vi "0-Write MDF.vi"(3 "error in":errorcluster, 4 "Global No Sail Circles":T2[](array[typedef]), 5 "Missions (Object Array)":refnum<class "GenericMission.lvclass">[](array[class])) -> (0 "error out":errorcluster)   [LabVIEW 2011]
doc: "Saves a MDF (Mission Definition File) to be later opened by 0-Read MDF.vi. MDF contains mission data: currently only a list of waypoints. The file uses the LabVIEW XML Schema."
uses:
  2-Think/2 Classes/Missions/GenericMission/GenericMission.lvclass
  2-Think/2 Typedefs/UTM Circle.ctl
  0 Typedefs/MDF data cluster.ctl
panel:
  out "MDF data cluster":T1
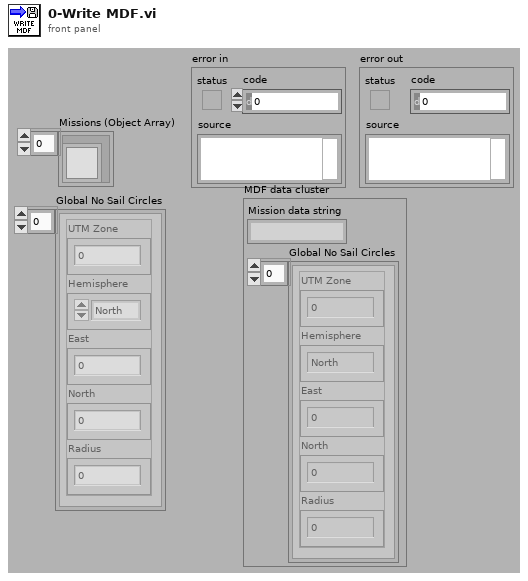
[diagram p1: front panel]
types:
  T1 = typedef "MDF data cluster.ctl" = cluster{"Mission data string":string, "Global No Sail Circles":T2[]}
  T2 = typedef "UTM Circle.ctl" = cluster{"UTM Zone":dbl, "Hemisphere":enum16{"North", "South"}, "East":dbl, "North":dbl, "Radius":dbl}
  T3 = cluster{"data string":string, "Global No Sail Circles":T2[]}
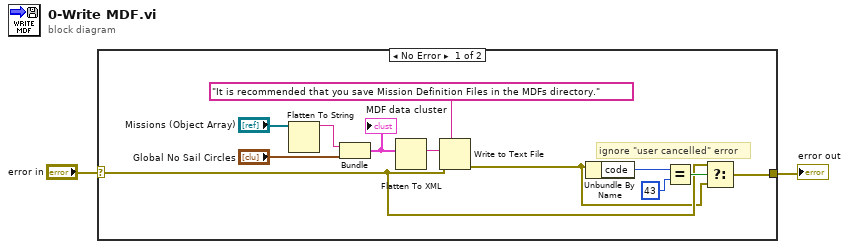
[diagram p0: block diagram]
diagram:
  n1 = case shown="No Error" "error in" {
    selector: "error in" -> [w9 w15]
    tunnel: [w7 w15] -> w1
    frame No Error {
      # "ignore \"user cancelled\" error"
      n2 = Flatten To String(anything="Missions (Object Array)") -> (data string=w5:string)  [unwired: 3 in, 2 out]
      n3 = Bundle("data string"=w5, "Global No Sail Circles"="Global No Sail Circles") -> (w6:T3)  [unwired: 1 in]
      "MDF data cluster" <- w6
      n4 = Flatten To XML(anything=w6) -> (xml string=w14:string)
      n5 = Write to Text File(prompt (Choose or enter file path)="It is recommended that you save Mission Definition Files in the MDFs directory.", text=w14, error in=w9) -> (error out=w8:errorcluster)  [unwired: 1 in, 2 out]
      n6 = Unbundle By Name(w8) -> ("code"=w12:i32)
      n7 = Equal?(x=w12, y=43 ("code")) -> (x = y?=w10:bool)
      n8 = Select(t=w9, s=w10, f=w8) -> (s? t:f=w7:errorcluster)
    }
    frame Error {
    }
  }
  "error out" <- w1
